vi "Do.vi"(8 "error in (no error)":errorcluster, 10 "Group Sizes":i64[](array[numeric]), 11 "Proto in":refnum<class "Group.lvclass">) -> (0 "error out":errorcluster, 2 "Arrangements":u64, 3 "Proto out":refnum<class "Group.lvclass">)   [LabVIEW 2020, in "Group.lvclass"]
uses:
  Group.lvclass
  Group.lvclass/Group.ctl
panel:
  out "Vaqlid?":bool
  in  "offset (0)":i32
  out "Array":string[](array[string])
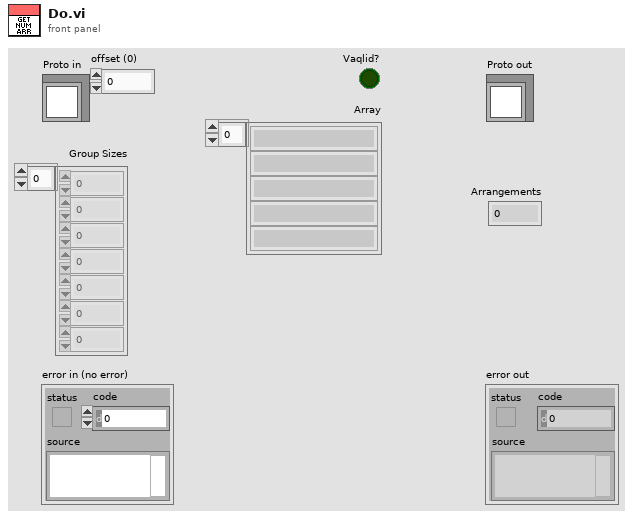
[diagram p1: front panel]
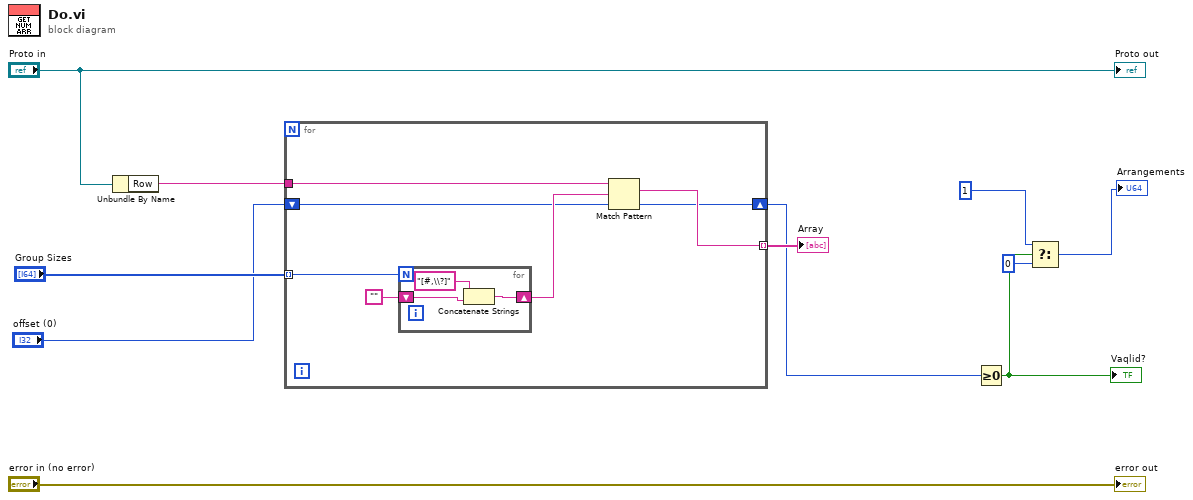
[diagram p0: block diagram]
diagram:
  n1 = Unbundle By Name("Proto in") -> ("Row"=w6:string)
  n2 = for {
    tunnel: "Group Sizes" -> [w16] mode=indexing
    tunnel: [w17] -> w8 mode=indexing
    tunnel: w6 -> [w18]
    shift-right: [w12] -> w5
    shift-left: "offset (0)" -> [w13]
    n3 = for {
      N: w16 -> [_]
      shift-right: [w20] -> w14
      shift-left: "" ("format string") -> [w19]
      n4 = Concatenate Strings("[#,\\?]" ("format string"), w19) -> (w20:string)
    }
    n5 = Match Pattern(string=w18, regular expression=w14, offset (0)=w13) -> (match substring=w17:string, offset past match=w12:i32)  [unwired: 2 out]
  }
  "Array" <- w8
  n6 = Greater Or Equal To 0?(x=w5) -> (x >= 0?=w4:bool)
  "Vaqlid?" <- w4
  n7 = Select(t=u64 1 ("Arrangements"), s=w4, f=u64 0) -> (s? t:f=→"Arrangements":u64)
  "error out" <- "error in (no error)"
  "Proto out" <- "Proto in"
